vi "Untitled 1.vi"() -> ()   [LabVIEW 2014]
panel:
  in  "1":dbl
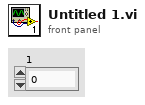
[diagram p1: front panel]
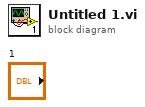
[diagram p0: block diagram]
diagram:
